vi "Run_Gnuplot_Script.vi"(0 "OutputType":enum16{"PDF", "PNG-ReportStyle"}(ring), 1 "logfileName":string, 2 "targetFile":path) -> ()   [LabVIEW 2021]
panel:
  out "stdErr":string
  out "stdOut":string
  out "error out":errorcluster
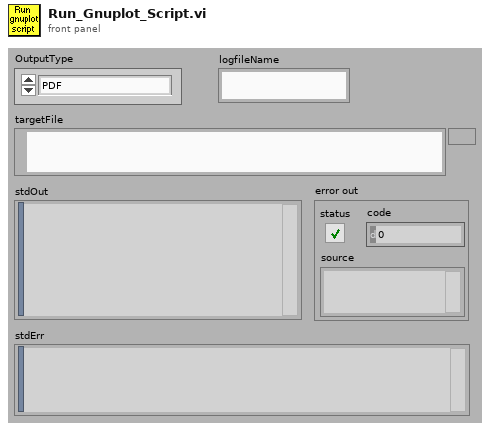
[diagram p1: front panel]
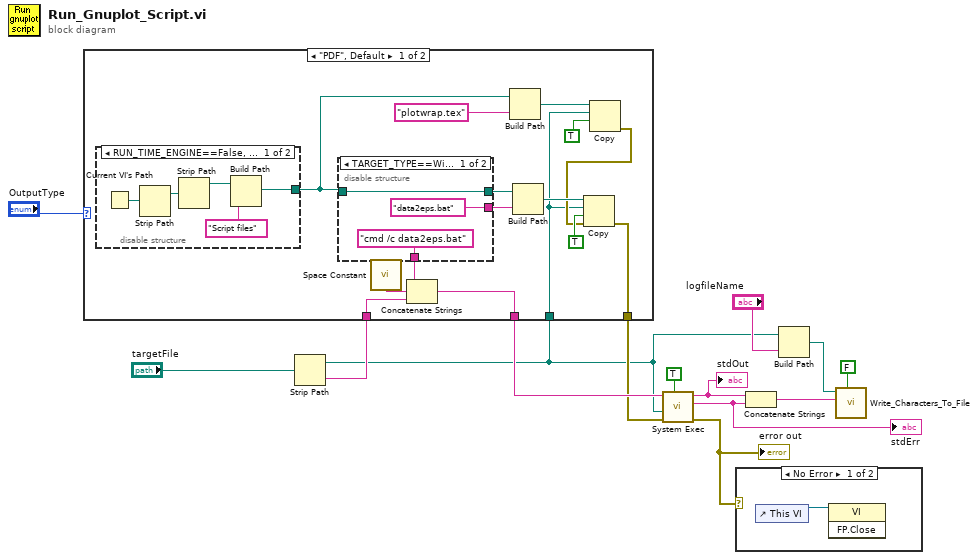
[diagram p0: block diagram]
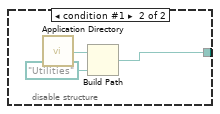
[diagram p3: hidden frame]
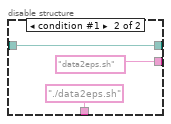
[diagram p4: hidden frame]
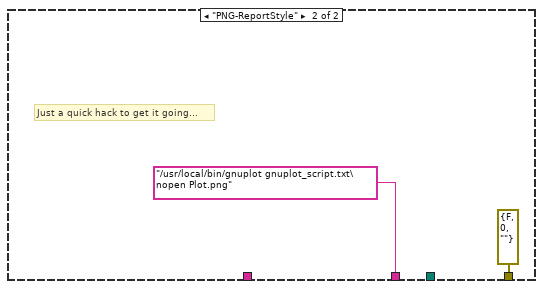
[diagram p5: hidden frame]
diagram:
  n1 = Strip Path(path="targetFile") -> (stripped path=w6:path, name=w9:string)
  n2 = case shown="\"PDF\", Default" "OutputType" {
    tunnel: [w28 "/usr/local/bin/gnuplot gnuplot_script.txt\nopen Plot.png"] -> w10
    tunnel: w9 -> [w24 _]
    tunnel: [w23 errorcluster {"status"=FALSE, "code"=0, "source"=""} ("error out")] -> w8
    tunnel: w6 -> [w15 _]
    frame "PDF", Default {
      n3 = disable-structure shown="RUN_TIME_ENGINE==False, Default" {
        disable-tunnel: [w31 w35] -> w18
        frame condition #0 (active) {
          n4 = Current VI's Path() -> (path=w34:path)
          n5 = Strip Path(path=w34) -> (stripped path=w33:path)  [unwired: 1 out]
          n6 = Strip Path(path=w33) -> (stripped path=w30:path)  [unwired: 1 out]
          n7 = Build Path(base path=w30, name or relative path="Script files") -> (appended path=w31:path)
        }
        frame condition #1 {
          n8 = call <vilib>:"Application Directory.vi"() -> ("Application Directory"=w37:path)
          n9 = Build Path(base path=w37, name or relative path=path "Utilities") -> (appended path=w35:path)
        }
      }
      n10 = disable-structure shown="TARGET_TYPE==Windows" {
        disable-tunnel: w18 -> [w38 w43]
        disable-tunnel: [w38 w43] -> w27
        disable-tunnel: ["data2eps.bat" "data2eps.sh"] -> w26
        disable-tunnel: ["cmd /c data2eps.bat" "./data2eps.sh"] -> w25
        frame condition #0 (active) {
        }
        frame condition #1 {
        }
      }
      n11 = call <vilib>:"Space Constant.vi"() -> ("String"=w29:string)
      n12 = Concatenate Strings(w25, w29, w24) -> (w28:string)
      n13 = Build Path(base path=w18, name or relative path="plotwrap.tex") -> (appended path=w20:path)
      n14 = Build Path(base path=w27, name or relative path=w26) -> (appended path=w21:path)
      n15 = Copy(9:TRUE ("overwrite (F)"), 10:w15, 11:w20) -> (0:w16:errorcluster)  [unwired: 1 in, 3 out]
      n16 = Copy(8:w16, 9:TRUE ("overwrite (F)"), 10:w15, 11:w21) -> (0:w23:errorcluster)  [unwired: 3 out]
    }
    frame "PNG-ReportStyle" {
      # "Just a quick hack to get it going..."
    }
  }
  n17 = call <vilib>:"System Exec.vi"("wait until completion? (T)"=TRUE, "error in (no error)"=w8, "working directory"=w6, "command line"=w10) -> ("error out"=w3:errorcluster, "standard error"=w1:string, "standard output"=w2:string)  [unwired: 2 in, 3 out]
  "error out" <- w3
  "stdOut" <- w2
  "stdErr" <- w1
  n18 = case shown="No Error" w3 {
    frame No Error {
      n19 = control-ref of="This VI"() -> (w46:refnum<vi>)
      n20 = invoke class="VI" method="FP.Close"(reference=w46) -> ()  [unwired: 2 in, 3 out]
    }
    frame Error {
    }
  }
  n21 = Concatenate Strings(w2, w1) -> (w7:string)
  n22 = Build Path(base path=w6, name or relative path="logfileName") -> (appended path=w13:path)
  n23 = call "Write_Characters_To_File.vi"("file path (dialog if empty)"=w13, "advisory dialog? (display:T)"=FALSE, "character string"=w7) -> ()  [unwired: 2 in, 4 out]
